vi "Channel.BuildDisplayedName.vi"(11 "Path":string) -> (3 "Formated Path":string)   [LabVIEW 2013, in "Simple Sequence Editor.lvlib"]
uses:
  Simple Sequence Editor.lvlib
  NationalInstruments.VeriStand
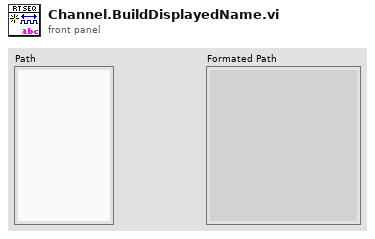
[diagram p1: front panel]
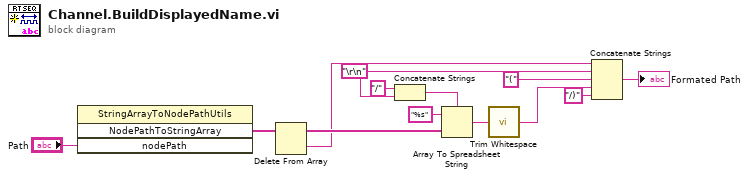
[diagram p0: block diagram]
diagram:
  w11 = "\r\n"
  n1 = invoke class="StringArrayToNodePathUtils" method="NodePathToStringArray"("nodePath"="Path") -> ("NodePathToStringArray"=w6:string[])  [unwired: 3 in, 3 out]
  n2 = Delete From Array(array=w6) -> (deleted portion=w7:string, array with subset deleted=w8:string[])  [unwired: 2 in]
  n3 = Concatenate Strings("/" ("string"), w11) -> (w10:string)
  n4 = Array To Spreadsheet String(delimiter (Tab)=w10, array=w8, 3:"%s" ("format string")) -> (spreadsheet string=w5:string)
  n5 = call <vilib>:"Trim Whitespace.vi"("string"=w5) -> ("trimmed string"=w3:string)  [unwired: 1 in]
  n6 = Concatenate Strings(w7, w11, "(" ("string"), w3, "/)" ("string")) -> (→"Formated Path":string)
